vi "Ref.vi"(7 "Event Actor in":refnum<class "Event Actor.lvclass">, 11 "Ref in":refnum<class "Ref.lvclass">) -> (5 "Event Actor out":refnum<class "Event Actor.lvclass">)   [LabVIEW 2021, in "Ref.lvclass"]
uses:
  Ref.lvclass
  Event Actor/Event Actor.lvclass
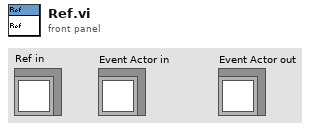
[diagram p1: front panel]
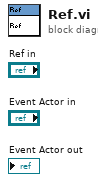
[diagram p0: block diagram]
diagram:
